vi "exp histogram circular.vi"(8 "amplitude":dbl format="%#_13g", 9 "tau":dbl format="%#_13g", 10 "t0":dbl, 11 "bin number":dbl[](array[numeric])) -> (3 "hist prediction":dbl[](array[numeric]))   [LabVIEW 2017]
panel:
  out "sum":dbl
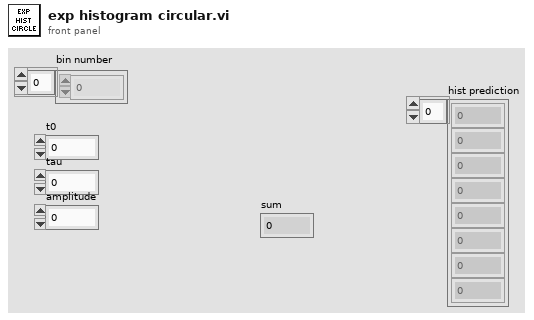
[diagram p1: front panel]
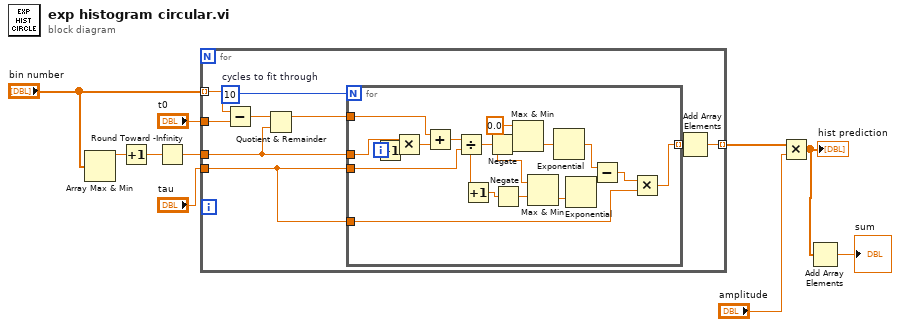
[diagram p0: block diagram]
diagram:
  n1 = Array Max & Min(array="bin number") -> (max value=w5:dbl)  [unwired: 3 out]
  n2 = Increment(x=w5) -> (x+1=w4:dbl)
  n3 = Round Toward -Infinity(1:w4) -> (0:w3:dbl)
  n4 = for {
    tunnel: "t0" -> [w19]
    tunnel: "tau" -> [w11]
    tunnel: [w14] -> w8 mode=indexing
    tunnel: "bin number" -> [w13] mode=indexing
    tunnel: w3 -> [w12]
    w17 = 10  # cycles to fit through
    n5 = Subtract(x=w13, y=w19) -> (x-y=w18:dbl)
    n6 = Quotient & Remainder(x=w18, y=w12) -> (x-y*floor(x/y)=w16:dbl)  [unwired: 1 out]
    n7 = for {
      N: w17 -> [_]
      tunnel: w16 -> [w37]
      tunnel: w12 -> [w35]
      tunnel: w11 -> [w33]
      tunnel: [w24] -> w15 mode=indexing
      tunnel: w11 -> [w25]
      i -> [w36]
      w22 = 0.0 ("x")
      n8 = Decrement(x=w36) -> (x-1=w20:i32)
      n9 = Multiply(x=w35, y=w20) -> (x*y=w34:dbl)
      n10 = Add(x=w37, y=w34) -> (x+y=w38:dbl)
      n11 = Divide(x=w38, y=w33) -> (x/y=w30:dbl)
      n12 = Increment(x=w30) -> (x+1=w29:dbl)
      n13 = Negate(x=w30) -> (-x=w32:dbl)
      n14 = Negate(x=w29) -> (-x=w23:dbl)
      n15 = Max & Min(x=w22, y=w32) -> (min(x,y)=w31:dbl)  [unwired: 1 out]
      n16 = Max & Min(x=w22, y=w23) -> (min(x,y)=w21:dbl)  [unwired: 1 out]
      n17 = Exponential(1:w31) -> (0:w28:dbl)
      n18 = Exponential(1:w21) -> (0:w27:dbl)
      n19 = Subtract(x=w28, y=w27) -> (x-y=w26:dbl)
      n20 = Multiply(x=w26, y=w25) -> (x*y=w24:dbl)
    }
    n21 = Add Array Elements(numeric array=w15) -> (sum=w14:dbl)
  }
  n22 = Multiply(x=w8, y="amplitude") -> (x*y=w2:dbl[])
  "hist prediction" <- w2
  n23 = Add Array Elements(numeric array=w2) -> (sum=→"sum":dbl)
